vi "Replace Backslash.vi"(11 "Barcode":string) -> (3 "连接的字符串":string)   [LabVIEW 2017, in "SQLite.lvclass"]
uses:
  SQLite.lvclass
panel:
  out "无符号字节数组":u8[](array[numeric])
  out "子字符串之后":string
  # "03210L817010000075*1008025-A401/D****-"
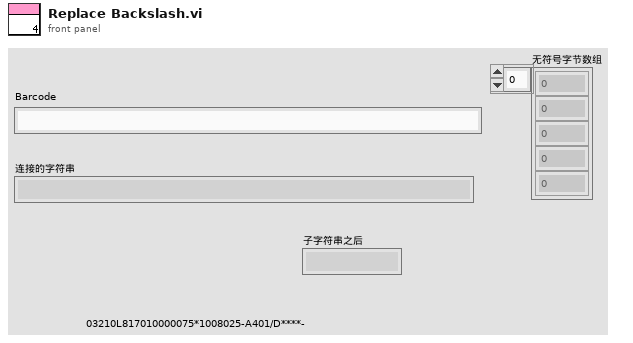
[diagram p1: front panel]
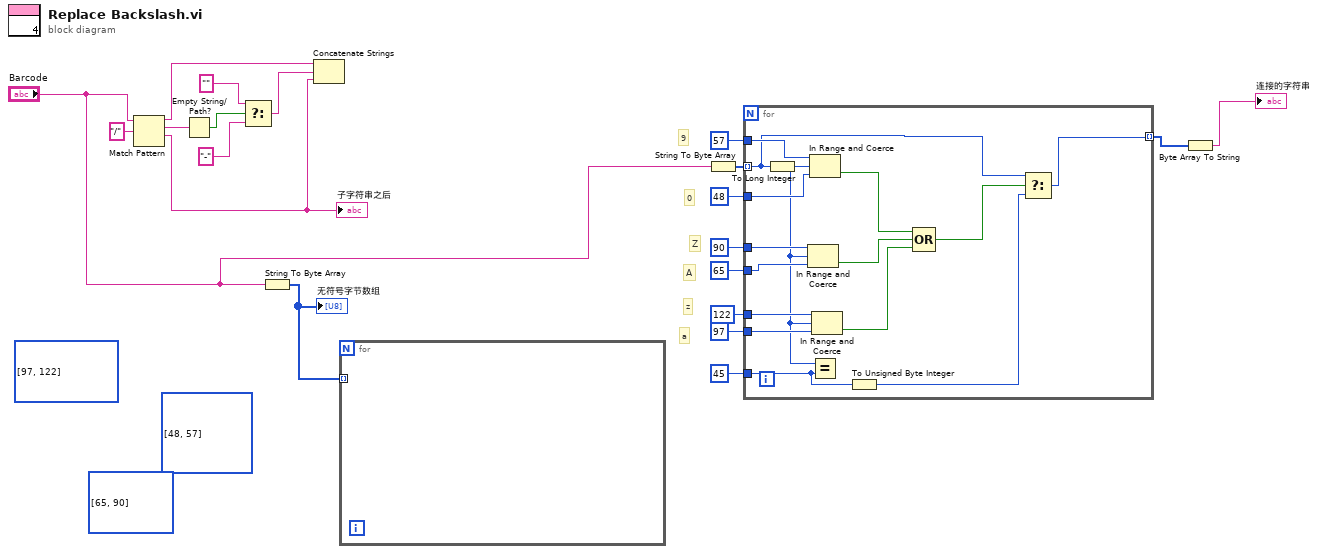
[diagram p0: block diagram]
diagram:
  (unwired) u8[] [97, 122] ("无符号字节数组")
  (unwired) u8[] [65, 90] ("无符号字节数组")
  (unwired) u8[] [48, 57] ("无符号字节数组")
  # "9"
  # "0"
  # "Z"
  # "A"
  # "z"
  # "a"
  n1 = Match Pattern(string="Barcode", regular expression="/" ("正则表达式")) -> (before substring=w19:string, match substring=w17:string, after substring=w18:string)  [unwired: 1 in, 1 out]
  "子字符串之后" <- w18
  n2 = Empty String/Path?(string/path=w17) -> (empty?=w16:bool)
  n3 = Select(t="" ("子字符串之后"), s=w16, f="-") -> (s? t:f=w13:string)
  n4 = String To Byte Array(string="Barcode") -> (unsigned byte array=w12:u8[])
  "无符号字节数组" <- w12
  n5 = Concatenate Strings(w19, w13, w18) -> ()  [unwired: 1 out]
  n6 = for {
    tunnel: w12 -> [_] mode=indexing
  }
  n7 = String To Byte Array(string="Barcode") -> (unsigned byte array=w9:u8[])
  n8 = for {
    tunnel: w9 -> [w22] mode=indexing
    tunnel: 48 ("lower limit") -> [w35]
    tunnel: 57 ("upper limit") -> [w34]
    tunnel: 90 ("upper limit") -> [w33]
    tunnel: 65 ("lower limit") -> [w32]
    tunnel: 122 ("upper limit") -> [w31]
    tunnel: 97 ("lower limit") -> [w30]
    tunnel: 45 ("lower limit") -> [w24]
    tunnel: [w21] -> w2 mode=indexing
    n9 = To Long Integer(number=w22) -> (32bit integer=w29:i32)
    n10 = In Range and Coerce(upper limit=w33, x=w29, lower limit=w32) -> (In Range?=w28:bool)  [unwired: 1 out]
    n11 = In Range and Coerce(upper limit=w34, x=w29, lower limit=w35) -> (In Range?=w26:bool)  [unwired: 1 out]
    n12 = Equal?(x=w29, y=w24) -> ()  [unwired: 1 out]
    n13 = In Range and Coerce(upper limit=w31, x=w29, lower limit=w30) -> (In Range?=w27:bool)  [unwired: 1 out]
    n14 = To Unsigned Byte Integer(number=w24) -> (unsigned 8bit integer=w23:u8)
    n15 = Compound Arithmetic op=OR(w26, w28, w27) -> (w25:bool)
    n16 = Select(t=w22, s=w25, f=w23) -> (s? t:f=w21:u8)
  }
  n17 = Byte Array To String(unsigned byte array=w2) -> (string=→"连接的字符串":string)
